vi "SetDataFolder.vi"(0 "User Data Folder":path, 5 "error in (no error)":errorcluster) -> (14 "Environment":refnum<k24>, 15 "UserDataFolder":string="C:\\ProgramData\\LcWebVIEW", 16 "Error Message":string, 19 "error out":errorcluster)   [LabVIEW 2019, in "LcWebView.lvclass"]
uses:
  LcWebView.lvclass
  C:/Projects/WebView2/LcWebView/data/Microsoft.Web.WebView2.Core.dll
  <vilib>/Utility/sysdir.llb/System Directory Type.ctl
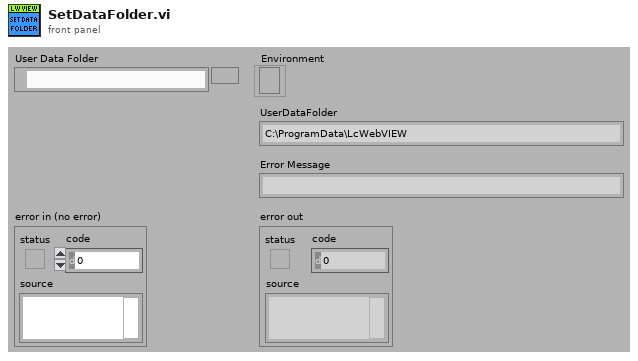
[diagram p1: front panel]
types:
  T1 = typedef "System Directory Type.ctl" = i32
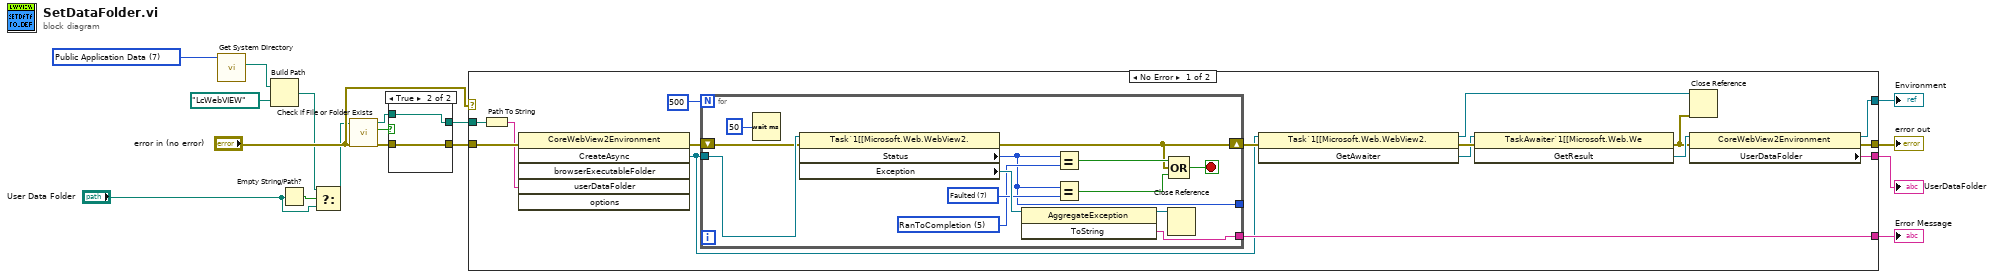
[diagram p0: block diagram]
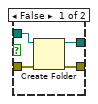
[diagram p2: hidden frame]
diagram:
  w13 = T1 7 items=["User Home"=0, "User Desktop"=1, "User Documents"=2, "User Application Data"=3, "User Preferences"=4, "User Temporary"=5, "Public Documents"=6, "Public Application Data"=7, "Public Preferences"=8, "Public Cache"=13, "System Core Libraries"=9, "System Installed Libraries"=10, "Application Files"=11, "Boot Volume Root"=12] ("system directory type")
  n1 = call <vilib>:"Get System Directory.vi"("system directory type"=w13) -> ("system directory"=w14:path)  [unwired: 10 in]
  n2 = Build Path(base path=w14, name or relative path=path "LcWebVIEW") -> (appended path=w2:path)
  n3 = Empty String/Path?(string/path="User Data Folder") -> (empty?=w4:bool)
  n4 = Select(t=w2, s=w4, f="User Data Folder") -> (s? t:f=w1:path)
  n5 = call <vilib>:"Check if File or Folder Exists.vi"("error in (no error)"="error in (no error)", "path"=w1) -> ("error out"=w17:errorcluster, "file or folder exists?"=w15:bool, "dup path"=w16:path)  [unwired: 7 in]
  n6 = case shown="True" w15 {
    tunnel: w16 -> [w21 w22]
    tunnel: w17 -> [w20 w23]
    tunnel: [w19 w23] -> w11
    tunnel: [w18 w22] -> w10
    frame False {
      n7 = Create Folder(path (use dialog)=w21, error in=w20) -> (created path=w18:path, error out=w19:errorcluster)  [unwired: 1 in, 1 out]
    }
    frame True {
    }
  }
  n8 = case shown="No Error" "error in (no error)" {
    selector: "error in (no error)" -> [_ w53]
    tunnel: w11 -> [w39 _]
    tunnel: w10 -> [w38 _]
    tunnel: [w25 w53] -> w9
    tunnel: [w36 _] -> w8
    tunnel: [w35 _] -> w7
    tunnel: [w24 _] -> w6
    frame No Error {
      n9 = Path To String(path=w38) -> (string=w37:string)
      n10 = invoke class="CoreWebView2Environment" method="CreateAsync"(error in=w39, "userDataFolder"=w37) -> (error out=w33:errorcluster, "CreateAsync"=w30:refnum<k24>)  [unwired: 4 in, 4 out]
      n11 = for {
        N: 500 -> [_]
        tunnel: w30 -> [w52]
        shift-right: [w45] -> w31
        shift-left: w33 -> [w51]
        tunnel: [w42] -> _
        tunnel: [w48] -> w35
        stop <- w43 stop-if-true
        w47 = 5 items=["Created", "WaitingForActivation", "WaitingToRun", "Running", "WaitingForChildrenToComplete", "RanToCompletion", "Canceled", "Faulted"] ("Status")
        w49 = 7 items=["Created", "WaitingForActivation", "WaitingToRun", "Running", "WaitingForChildrenToComplete", "RanToCompletion", "Canceled", "Faulted"] ("Status")
        n12 = Wait (ms)(milliseconds to wait=u32 50) -> ()  [unwired: 1 out]
        n13 = property class="Task`1[[Microsoft.Web.WebView2."(reference=w52, error in=w51) -> (error out=w45:errorcluster, "Status"=w42:i32, "Exception"=w50:refnum<k24>)  [unwired: 1 out]
        n14 = invoke class="AggregateException" method="ToString"(reference=w50) -> (reference out=w41:refnum<k24>, "ToString"=w48:string)  [unwired: 2 in, 1 out]
        n15 = Equal?(x=w42, y=w47) -> (x = y?=w46:bool)
        n16 = Equal?(x=w42, y=w49) -> (x = y?=w44:bool)
        n17 = Close Reference(reference=w41) -> ()  [unwired: 1 in, 1 out]
        n18 = Compound Arithmetic op=OR(w46, w45, w44) -> (w43:bool)
      }
      n19 = invoke class="Task`1[[Microsoft.Web.WebView2." method="GetAwaiter"(reference=w30, error in=w31) -> (reference out=w27:refnum<k24>, error out=w32:errorcluster, "GetAwaiter"=w28:refnum<k24>)  [unwired: 1 in]
      n20 = invoke class="TaskAwaiter`1[[Microsoft.Web.We" method="GetResult"(reference=w28, error in=w32) -> (error out=w26:errorcluster, "GetResult"=w29:refnum<k24>)  [unwired: 1 in, 1 out]
      n21 = Close Reference(reference=w27, error in (no error)=w26) -> ()  [unwired: 1 out]
      n22 = property class="CoreWebView2Environment"(reference=w29, error in=w26) -> (reference out=w24:refnum<k24>, error out=w25:errorcluster, "UserDataFolder"=w36:string)
    }
    frame Error {
    }
  }
  "error out" <- w9
  "UserDataFolder" <- w8
  "Error Message" <- w7
  "Environment" <- w6
